vi "Download Recipe_galil.vi"(8 "error in (no error)":errorcluster, 10 "Parameter":T1, 11 "Programing Logic in":refnum<class "Programing Logic.lvclass">) -> (0 "error out":errorcluster, 3 "Programing Logic out":refnum<class "Programing Logic.lvclass">)   [LabVIEW 2014, in "Programing Logic.lvclass"]
uses:
  Programing Logic.lvclass
  Programing Logic.lvclass/Programing Logic.ctl
panel:
  out "concatenated string 2":string
  out "concatenated string":string
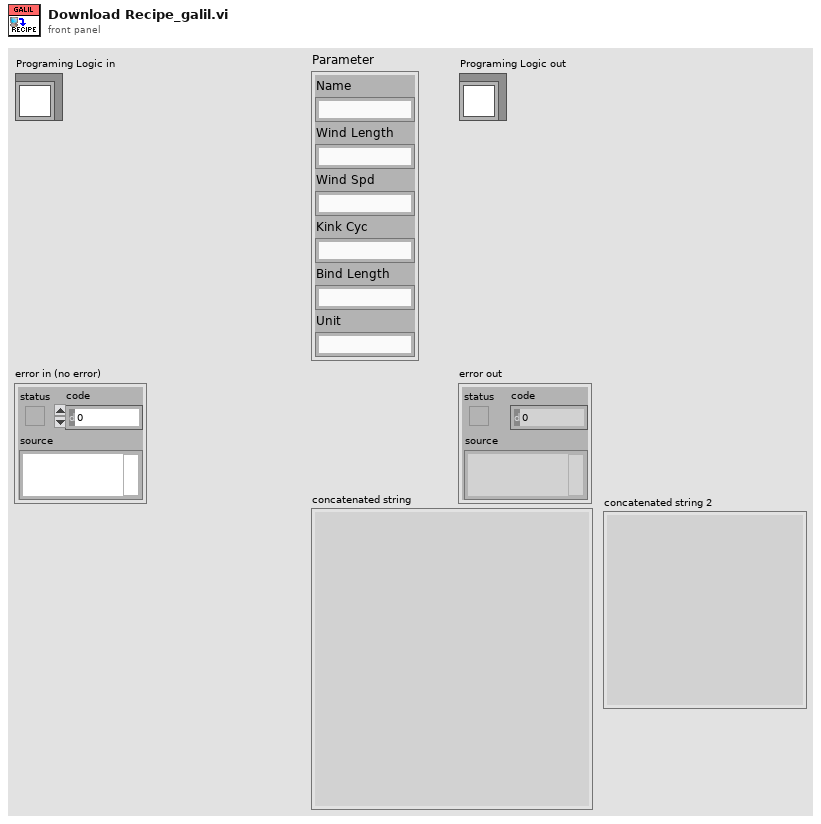
[diagram p1: front panel]
types:
  T1 = cluster{"Name":string, "Wind Length":string, "Wind Spd":string, "Kink Cyc":string, "Bind Length":string, "Unit":string}
  T2 = cluster{"Wind Spd":string, "Wind Length":string, "Unit":string}
  T3 = cluster{"Kink Cyc":string, "Bind Length":string, "Unit":string}
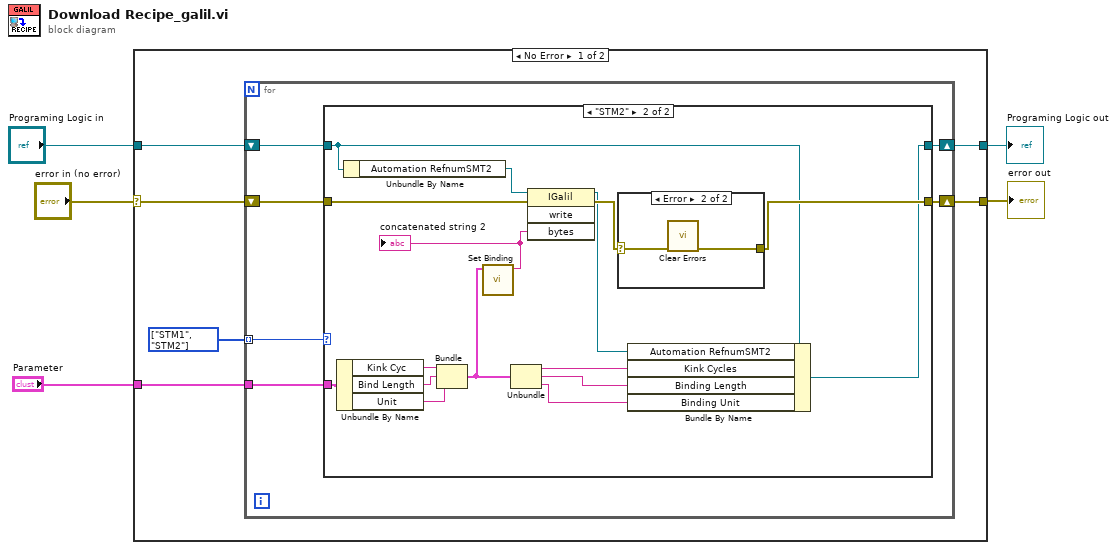
[diagram p0: block diagram]
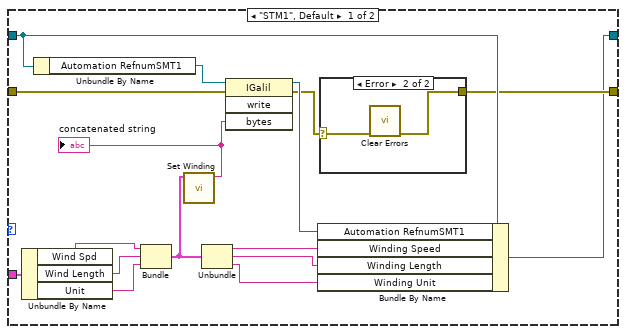
[diagram p2: hidden frame]
diagram:
  n1 = case shown="No Error" "error in (no error)" {
    selector: "error in (no error)" -> [w7 w57]
    tunnel: [w6 w57] -> w4
    tunnel: [w9 w56] -> w2
    tunnel: "Programing Logic in" -> [w10 w56]
    tunnel: "Parameter" -> [w8 _]
    frame No Error {
      w11 = enum16{"STM1", "STM2"}[] [enum."STM1", enum."STM2"] items=["STM1", "STM2"]
      n2 = for {
        tunnel: w11 -> [w17] mode=indexing
        shift-right: [w15] -> w9
        shift-left: w10 -> [w16]
        tunnel: w8 -> [w14]
        shift-right: [w12] -> w6
        shift-left: w7 -> [w13]
        n3 = case shown="\"STM2\"" w17 {
          tunnel: w16 -> [w30 w48]
          tunnel: [w22 w46] -> w15
          tunnel: w14 -> [w33 w45]
          tunnel: w13 -> [w31 w51]
          tunnel: [w23 w49] -> w12
          frame "STM1", Default {
            n4 = Unbundle By Name(w33) -> ("Wind Spd"=w28:string, "Wind Length"=w29:string, "Unit"=w27:string)
            n5 = Unbundle By Name(w30) -> ("Automation RefnumSMT1"=w32:refnum<k7>)
            n6 = Bundle("Wind Spd"=w28, "Wind Length"=w29, "Unit"=w27) -> (w21:T2)  [unwired: 1 in]
            n7 = call "Set Winding.vi"("Recipes.Winding"=w21) -> ("concatenated string"=w26:string)  [unwired: 10 in]
            "concatenated string" <- w26
            n8 = Unbundle(w21) -> ("Wind Spd"=w20:string, "Wind Length"=w19:string, "Unit"=w18:string)
            n9 = invoke class="IGalil" method="write"(reference=w32, error in=w31, "bytes"=w26) -> (reference out=w25:refnum<k7>, error out=w24:errorcluster)  [unwired: 1 in, 2 out]
            n10 = Bundle By Name(cluster=w30, "Automation RefnumSMT1"=w25, "Winding Speed"=w20, "Winding Length"=w19, "Winding Unit"=w18) -> (w22:refnum<class "Programing Logic.lvclass">)
            n11 = case shown="Error" w24 {
              selector: w24 -> [w34 w36]
              tunnel: [w34 w35] -> w23
              frame No Error {
              }
              frame Error {
                n12 = call <vilib>:"Clear Errors.vi"("error in (no error)"=w36) -> ("error out"=w35:errorcluster)  [unwired: 5 in, 1 out]
              }
            }
          }
          frame "STM2" {
            n13 = Unbundle By Name(w45) -> ("Kink Cyc"=w44:string, "Bind Length"=w43:string, "Unit"=w42:string)
            n14 = Unbundle By Name(w48) -> ("Automation RefnumSMT2"=w52:refnum<k7>)
            n15 = Bundle("Kink Cyc"=w44, "Bind Length"=w43, "Unit"=w42) -> (w40:T3)  [unwired: 1 in]
            n16 = call "Set Binding.vi"("Recipes.Binding"=w40) -> ("concatenated string"=w41:string)  [unwired: 10 in]
            "concatenated string 2" <- w41
            n17 = Unbundle(w40) -> ("Kink Cyc"=w39:string, "Bind Length"=w38:string, "Unit"=w37:string)
            n18 = invoke class="IGalil" method="write"(reference=w52, error in=w51, "bytes"=w41) -> (reference out=w47:refnum<k7>, error out=w50:errorcluster)  [unwired: 1 in, 2 out]
            n19 = case shown="Error" w50 {
              selector: w50 -> [w53 w55]
              tunnel: [w53 w54] -> w49
              frame No Error {
              }
              frame Error {
                n20 = call <vilib>:"Clear Errors.vi"("error in (no error)"=w55) -> ("error out"=w54:errorcluster)  [unwired: 5 in, 1 out]
              }
            }
            n21 = Bundle By Name(cluster=w48, "Automation RefnumSMT2"=w47, "Kink Cycles"=w39, "Binding Length"=w38, "Binding Unit"=w37) -> (w46:refnum<class "Programing Logic.lvclass">)
          }
        }
      }
    }
    frame Error {
    }
  }
  "error out" <- w4
  "Programing Logic out" <- w2
